vi "LINX - PmodTMP3.vi"() -> ()   [LabVIEW 2020]
doc: "PmodTMP3\n\nThis example demonstrates how to read the angular velocity values from the PmodTMP3.\n\nInstructions:\n1. Select the COM Port associated with the LINX device\n2. Select the I2C Channel that the Pmod is connected to.\n3. Select the Slave Address for the Pmod (default 0x48 with all jumpers to ground)\n4. Select the desired resolution.\n5. Click the Run Arrow."
uses:
  vi.lib/MakerHub/LINX/Public/Utilities/Open Serial.vi
  vi.lib/MakerHub/LINX/Public/Sensors/Pmods/TMP3/PmodTMP3.lvlib
  vi.lib/MakerHub/LINX/LMH-LINX.lvlib
panel:
  out "Waveform Chart":dbl(graph)
  in  "Stop Button":bool
  out "Ambient Temperature (C)":dbl
  in  "Resolution":enum16{"0.5", "0.25", "0.125", "0.0625"}(ring)
  in  "Slave Address":T1(ring)
  in  "Serial Port":refnum<visa-resource-name>="N/A"
  in  "I2C Channel (0)":u8
  # "PmodTMP3\n\nThis example demonstrates how to read the angular velocity values from the PmodTMP3.\n\nInstructions:\n1. Select the COM Port associated with the LINX device\n2. Select the I2C Channel that the Pmod is connected to.\n3. Select the Slave Address for the Pmod (default 0x48 with all jumpers to ground)\n4. Select the desired resolution.\n5. Click the Run Arrow."
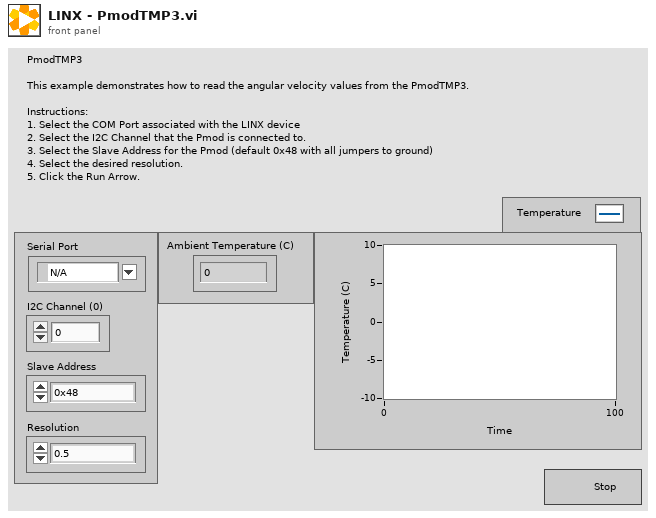
[diagram p1: front panel]
types:
  T1 = enum8{"0x48", "0x49", "0x4A", "0x4B", "0x4C", "0x4D", "0x4E", "0x4F"}
  T2 = typedef "LMH-LINX.lvlib/LINX Ref.ctl" = cluster{"IO":T3, "Interface":T4, "LINX Device Config":T5}
  T3 = typedef "LMH-LINX.lvlib/Platform.ctl" = enum16{"Remote", "Local"}
  T4 = typedef "LMH-LINX.lvlib/Interface.ctl" = enum16{"Serial", "TCP"}
  T5 = typedef "Device.lvlib/LINX Device Config.ctl" = cluster{"Interface":T4, "COM Port":refnum<visa-resource-name>, "TCP Configuration":T6, "Device Family":u8, "Device ID":u8, "Device Name":string, "TCP Ref":refnum<k5>, "Channels":T7}
  T6 = typedef "Device.lvlib/TCP Config.ctl" = cluster{"IP Address":string, "Port":u16}
  T7 = typedef "LMH-LINX.lvlib/Channels.ctl" = cluster{"DI":u8[], "DO":u8[], "AI":u8[], "AO":u8[], "PWM":u8[], "QE":u8[], "UART":u8[], "I2C 2":u8[], "SPI":u8[], "CAN":u8[], "Servo":u8[], "AI Ref (V)":dbl, "AI Resolution (Bits)":u8, "AO Ref (V)":dbl, "AO Resolution (Bits)":u8}
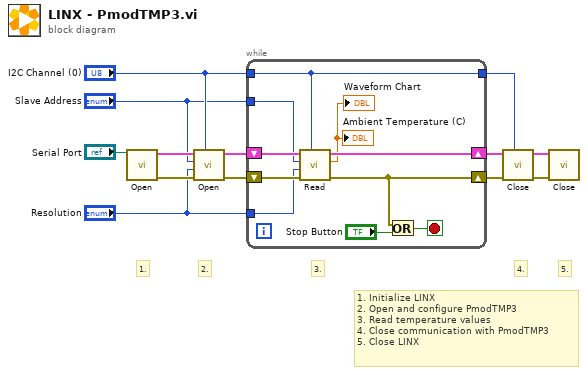
[diagram p0: block diagram]
diagram:
  # "1. Initialize LINX\n2. Open and configure PmodTMP3\n3. Read temperature values\n4. Close communication with PmodTMP3\n5. Close LINX"
  # "5."
  # "4."
  # "3."
  # "2."
  # "1."
  n1 = call-poly "Open.vi"("Serial Port"="Serial Port") -> ("Error Out"=w12:errorcluster, "LINX Resource"=w13:T2)  [unwired: 8 in, 1 out]
  n2 = call "Open.vi"("I2C Channel (0)"="I2C Channel (0)", "Error In"=w12, "Resolution"="Resolution", "Slave Address"="Slave Address", "LINX Resource"=w13) -> ("Error Out"=w11:errorcluster, "LINX Resource"=w10:T2)  [unwired: 4 in, 1 out]
  n3 = while {
    tunnel: "I2C Channel (0)" -> [w15]
    tunnel: "Slave Address" -> [w20]
    tunnel: "Resolution" -> [w19]
    shift-right: [w16] -> w8
    shift-left: w11 -> [w23]
    shift-right: [w21] -> w9
    shift-left: w10 -> [w22]
    tunnel: [w15] -> w1
    stop <- w18 stop-if-true
    n4 = call "Read.vi"("I2C Channel (0)"=w15, "Error In"=w23, "Resolution"=w19, "Slave Address"=w20, "LINX Resource"=w22) -> ("Error Out"=w16:errorcluster, "Ambient Temperature (C)"=→"Ambient Temperature (C)" →"Waveform Chart":dbl, "LINX Resource"=w21:T2)  [unwired: 4 in]
    n5 = Or(x=w16, y="Stop Button") -> (x .or. y?=w18:bool)
  }
  n6 = call "Close.vi"("I2C Channel (0)"=w1, "Error In"=w8, "LINX Resource"=w9) -> ("Error Out"=w7:errorcluster, "LINX Resource"=w6:T2)  [unwired: 7 in]
  n7 = call "Close.vi"("Error In"=w7, "LINX Resource"=w6) -> ()  [unwired: 9 in, 1 out]
